vi "Stop_Display.vi"(4 "Numeric":u32) -> (1 "Colors [4]":cluster{u32, u32}[](array[cluster]))   [LabVIEW 2019]
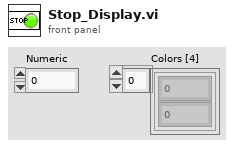
[diagram p1: front panel]
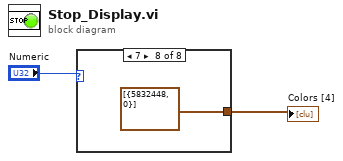
[diagram p0: block diagram]
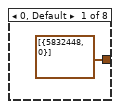
[diagram p2: hidden frame]
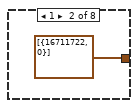
[diagram p3: hidden frame]
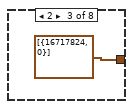
[diagram p4: hidden frame]
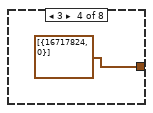
[diagram p5: hidden frame]
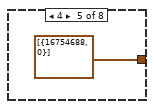
[diagram p6: hidden frame]
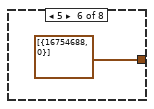
[diagram p7: hidden frame]
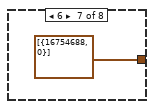
[diagram p8: hidden frame]
diagram:
  n1 = case shown="7" "Numeric" {
    tunnel: [cluster{u32, u32}[] [{5832448, 0}] ("Colors [4]") cluster{u32, u32}[] [{16711722, 0}] ("Colors [4]") cluster{u32, u32}[] [{16717824, 0}] ("Colors [4]") cluster{u32, u32}[] [{16717824, 0}] ("Colors [4]") cluster{u32, u32}[] [{16754688, 0}] ("Colors [4]") cluster{u32, u32}[] [{16754688, 0}] ("Colors [4]") cluster{u32, u32}[] [{16754688, 0}] ("Colors [4]") cluster{u32, u32}[] [{5832448, 0}] ("Colors [4]")] -> w2
    frame 0, Default {
    }
    frame 1 {
    }
    frame 2 {
    }
    frame 3 {
    }
    frame 4 {
    }
    frame 5 {
    }
    frame 6 {
    }
    frame 7 {
    }
  }
  "Colors [4]" <- w2
